vi "In Basic Series_.vi"(8 "2D sel":T2, 10 "1D sel":T2, 11 "E-Series Data":T3) -> (3 "In Basic?":T1)   [LabVIEW 2018]
uses:
  E-Series Reader/series data--cluster.ctl
  digit--enum.ctl
  In low series--cluster.ctl
  E-Series Reader/E-Series Reader.lvlib
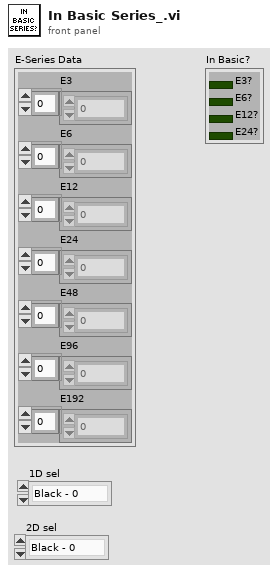
[diagram p1: front panel]
types:
  T1 = typedef "In low series--cluster.ctl" = cluster{"E3?":bool, "E6?":bool, "E12?":bool, "E24?":bool}
  T2 = typedef "digit--enum.ctl" = enum16{"Black - 0", "Brown - 1", "Red - 2", "Orange - 3", "Yellow - 4", "Green - 5", "Blue - 6", "Violet - 7", "Grey - 8", "White - 9"}
  T3 = typedef "E-Series Reader.lvlib/series data--cluster.ctl" = cluster{"E3":u16[], "E6":u16[], "E12":u16[], "E24":u16[], "E48":u16[], "E96":u16[], "E192":u16[]}
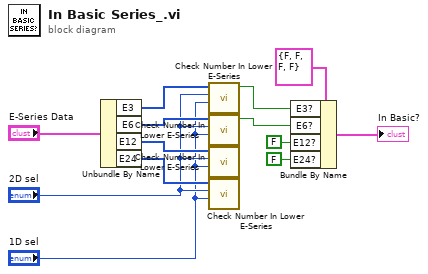
[diagram p0: block diagram]
diagram:
  n1 = Unbundle By Name("E-Series Data") -> ("E3"=w12:u16[], "E6"=w11:u16[], "E12"=w10:u16[], "E24"=w9:u16[])
  n2 = call "Check Number In Lower E-Series.vi"("1D sel"="1D sel", "2D sel"="2D sel", "E Serie"=w12) -> ("In Serie?"=w6:bool)  [unwired: 8 in]
  n3 = call "Check Number In Lower E-Series.vi"("1D sel"="1D sel", "2D sel"="2D sel", "E Serie"=w11) -> ("In Serie?"=w5:bool)  [unwired: 8 in]
  n4 = call "Check Number In Lower E-Series.vi"("1D sel"="1D sel", "2D sel"="2D sel", "E Serie"=w10) -> ()  [unwired: 8 in, 1 out]
  n5 = call "Check Number In Lower E-Series.vi"("1D sel"="1D sel", "2D sel"="2D sel", "E Serie"=w9) -> ()  [unwired: 8 in, 1 out]
  n6 = Bundle By Name(cluster=T1 {"E3?"=FALSE, "E6?"=FALSE, "E12?"=FALSE, "E24?"=FALSE} ("In Lower"), "E3?"=w6, "E6?"=w5, "E12?"=FALSE, "E24?"=FALSE) -> (→"In Basic?":T1)
